vi "GetType.vi"(8 "error in (no error)":errorcluster, 11 "Set Output Values Msg":refnum<class "Set Output Values Msg.lvclass">) -> (0 "error out":errorcluster, 2 "Data Sample":variant, 3 "Set Output Values Msg":refnum<class "Set Output Values Msg.lvclass">)   [LabVIEW 2020, in "BNT_DAQmx.lvlib" / "Set Output Values Msg.lvclass"]
uses:
  Set Output Values Msg.lvclass
  Set Output Values Msg.lvclass/Set Output Values Msg.ctl
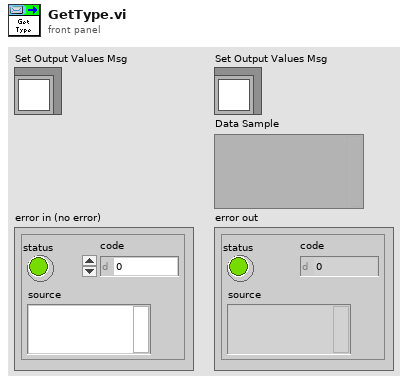
[diagram p1: front panel]
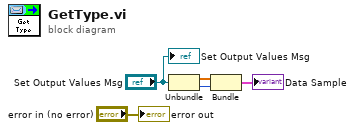
[diagram p0: block diagram]
diagram:
  n1 = Unbundle("Set Output Values Msg") -> (w2:dbl[], w1:i32)
  n2 = Bundle("Values"=w2, "Start Index"=w1) -> (→"Data Sample":cluster{"Values":dbl[], "Start Index":i32})  [unwired: 1 in]
  "error out" <- "error in (no error)"
  "Set Output Values Msg" <- "Set Output Values Msg"
